vi "PostionPaneViewScrollbars.vi"(8 "error in (no error)":errorcluster, 10 "Set Origin to ((0,0))":T1, 11 "vi path":path) -> (0 "error out":errorcluster)   [LabVIEW 2013]
doc: "Set VI pane scrollbar positions. Default is to place (0,0) (diamond on grid) at top left.\nTo use, pass \"Current VI Path.\""
uses:
  <vilib>/Utility/miscctls.llb/LVPointTypeDef.ctl
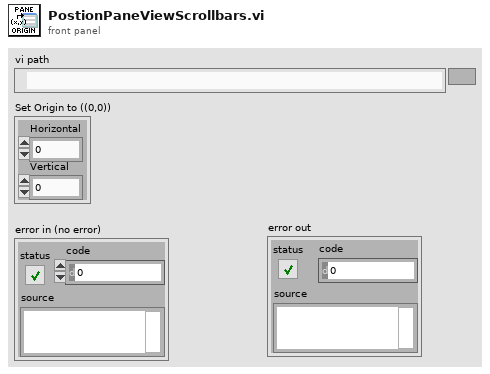
[diagram p1: front panel]
types:
  T1 = typedef "LVPointTypeDef.ctl" = cluster{"Horizontal":i16, "Vertical":i16}
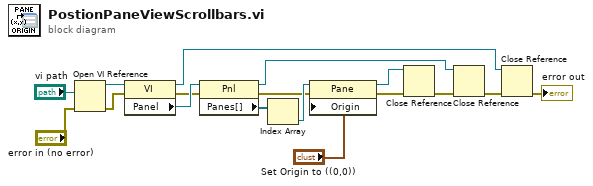
[diagram p0: block diagram]
diagram:
  n1 = Open VI Reference(vi path="vi path", error in (no error)="error in (no error)") -> (vi reference=w17:refnum<vi>, error out=w7:errorcluster)  [unwired: 4 in]
  n2 = property class="VI"(reference=w17, error in=w7) -> (reference out=w11:refnum<vi>, error out=w6:errorcluster, "Panel"=w16:refnum<vi>)
  n3 = property class="Pnl"(reference=w16, error in=w6) -> (reference out=w15:refnum<vi>, error out=w5:errorcluster, "Panes[]"=w13:refnum<vi>[])
  n4 = Index Array(array=w13) -> (element=w12:refnum<vi>)  [unwired: 1 in]
  n5 = property class="Pane"(reference=w12, error in=w5, "Origin"="Set Origin to ((0,0))") -> (reference out=w14:refnum<vi>, error out=w4:errorcluster)
  n6 = Close Reference(reference=w14, error in (no error)=w4) -> (error out=w3:errorcluster)
  n7 = Close Reference(reference=w15, error in (no error)=w3) -> (error out=w2:errorcluster)
  n8 = Close Reference(reference=w11, error in (no error)=w2) -> (error out=→"error out":errorcluster)
